vi "myRIO_BRig_RT__calc_laser_FPGA_N.vi"(0 "input_FPGA_ms2count":dbl, 5 "input_Tpeak":dbl, 7 "input_Freq":dbl, 9 "input_Tshutter":dbl, 11 "input_duration":u16) -> (4 "output_laser_Npeak":u32, 6 "output_laser_Nvalley":u32, 8 "output_laser_Nshutter":u32, 10 "output_laser_Nduration":u32, 15 "output_laser_Tduration":u16)   [LabVIEW 2014]
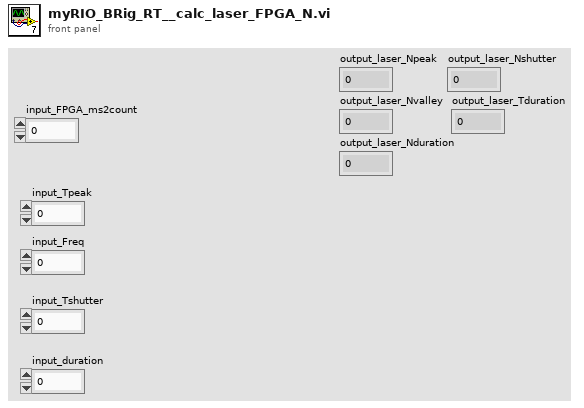
[diagram p1: front panel]
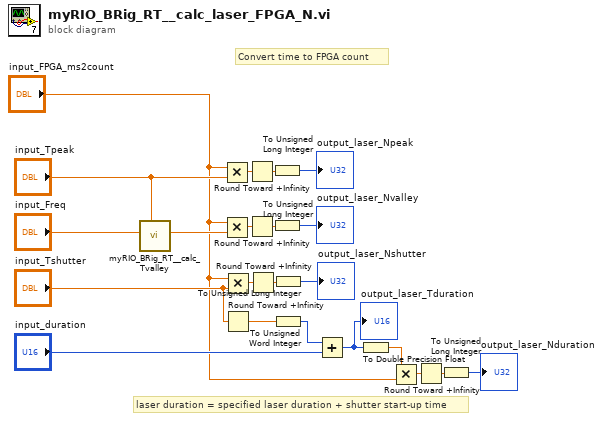
[diagram p0: block diagram]
diagram:
  # "laser duration = specified laser duration + shutter start-up time"
  # "Convert time to FPGA count"
  n1 = call "myRIO_BRig_RT__calc_Tvalley.vi"("input_peakWidth"="input_Tpeak", "input_freq"="input_Freq") -> ("output_Tvalley"=w13:dbl)  [unwired: 9 in]
  n2 = Multiply(x="input_FPGA_ms2count", y="input_Tpeak") -> (x*y=w16:dbl)
  n3 = Multiply(x="input_FPGA_ms2count", y=w13) -> (x*y=w18:dbl)
  n4 = Multiply(x="input_FPGA_ms2count", y="input_Tshutter") -> (x*y=w19:dbl)
  n5 = Round Toward +Infinity(x="input_Tshutter") -> (ceil(x): smallest int >= x=w21:dbl)
  n6 = Round Toward +Infinity(x=w16) -> (ceil(x): smallest int >= x=w15:dbl)
  n7 = Round Toward +Infinity(x=w18) -> (ceil(x): smallest int >= x=w17:dbl)
  n8 = Round Toward +Infinity(x=w19) -> (ceil(x): smallest int >= x=w20:dbl)
  n9 = To Unsigned Long Integer(number=w15) -> (unsigned 32bit integer=→"output_laser_Npeak":u32)
  n10 = To Unsigned Long Integer(number=w17) -> (unsigned 32bit integer=→"output_laser_Nvalley":u32)
  n11 = To Unsigned Long Integer(number=w20) -> (unsigned 32bit integer=→"output_laser_Nshutter":u32)
  n12 = To Unsigned Word Integer(number=w21) -> (unsigned 16bit integer=w8:u16)
  n13 = Add(x=w8, y="input_duration") -> (x+y=w1:u16)
  "output_laser_Tduration" <- w1
  n14 = To Double Precision Float(number=w1) -> (double precision float=w7:dbl)
  n15 = Multiply(x=w7, y="input_FPGA_ms2count") -> (x*y=w11:dbl)
  n16 = Round Toward +Infinity(x=w11) -> (ceil(x): smallest int >= x=w10:dbl)
  n17 = To Unsigned Long Integer(number=w10) -> (unsigned 32bit integer=→"output_laser_Nduration":u32)
